vi "Mike.vi"() -> ()   [LabVIEW 2013]
uses:
  <vilib>/Analysis/2dsp.llb/Real FFT.vi
  <instrlib>/niUSRP/niUSRP Fetch Rx Data (CDB).vi
  <vilib>/Analysis/NI_AALPro.lvlib
panel:
  out "Waveform Graph 3":dbl[](graph)
  out "Waveform Graph 2":dbl[][](graph)
  out "Waveform Graph":dbl[](graph)
  in  "stop":bool
  in  "RX number of samples":i64=100000
  out "RX coerced gain":dbl format="%#_6f"
  out "RX coerced IQ rate":dbl=100000.0 format="%#_6p"
  in  "RX gain":dbl format="%#_6f"
  in  "RX IQ rate":dbl=100000.0 format="%#_6p"
  in  "device names":refnum<k15>
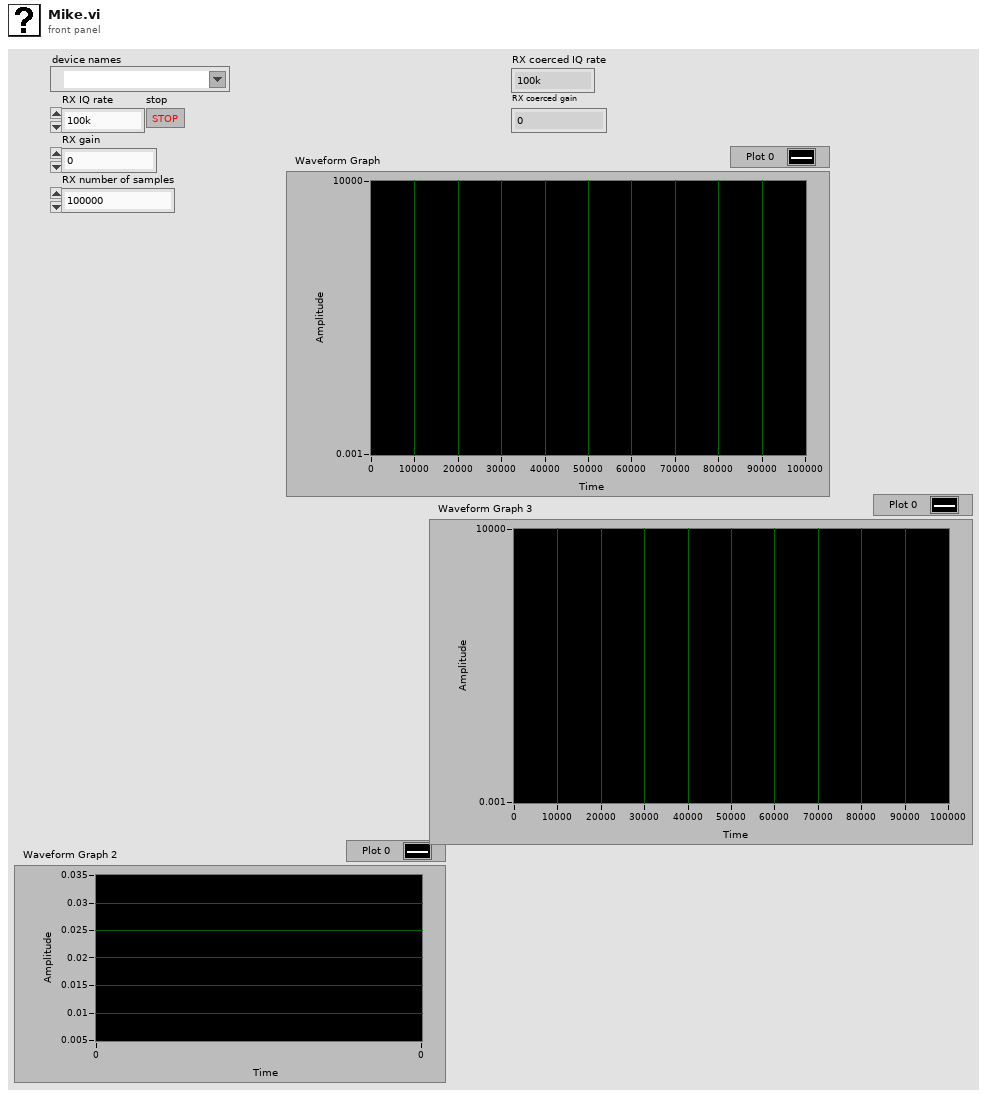
[diagram p1: front panel]
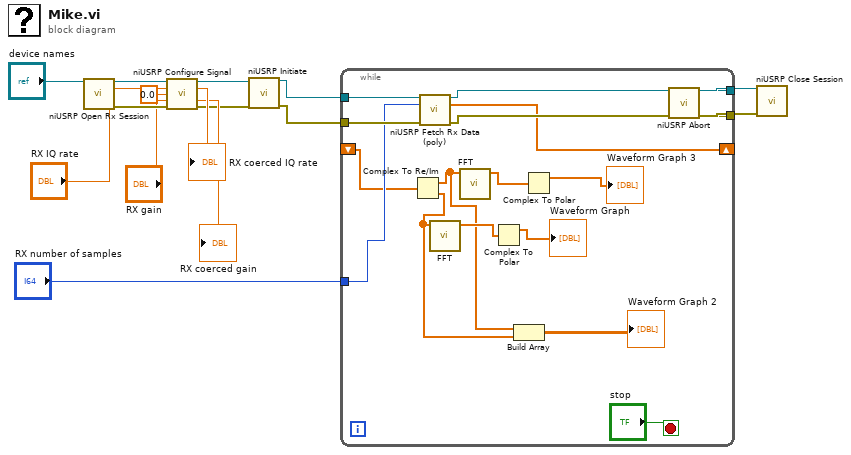
[diagram p0: block diagram]
diagram:
  n1 = call <instrlib>:"niUSRP Open Rx Session.vi"("device names"="device names") -> ("session handle out"=w16:refnum<k15>, "error out"=w14:errorcluster)  [unwired: 13 in]
  n2 = call <instrlib>:"niUSRP Configure Signal.vi"("session handle"=w16, "IQ rate"="RX IQ rate", "carrier frequency"=0.0, "gain"="RX gain", "error in (no error)"=w14) -> ("session handle out"=w3:refnum<k15>, "coerced IQ rate"=→"RX coerced IQ rate":dbl, "coerced gain"=→"RX coerced gain":dbl, "error out"=w2:errorcluster)  [unwired: 6 in, 1 out]
  n3 = call <instrlib>:"niUSRP Initiate.vi"("session handle"=w3, "error in (no error)"=w2) -> ("session handle out"=w4:refnum<k15>, "error out"=w8:errorcluster)  [unwired: 12 in]
  n4 = while {
    tunnel: w4 -> [w32]
    tunnel: w8 -> [w31]
    tunnel: [w30] -> w7
    tunnel: [w29] -> w6
    tunnel: "RX number of samples" -> [w26]
    shift-right: [w27] -> _
    shift-left: _ -> [w23]
    stop <- "stop" stop-if-true
    n5 = Complex To Re/Im(x + iy=w23) -> (x=w21:dbl[], y=w20:dbl[])
    n6 = call-poly <instrlib>:"niUSRP Fetch Rx Data (poly).vi"("session handle"=w32, "number of samples"=w26, "error in (no error)"=w31) -> ("session handle out"=w30:refnum<k15>, "data"=w27:cdb[], "error out"=w29:errorcluster)  [unwired: 9 in, 1 out]
    n7 = call-poly <vilib>:"FFT.vi"("X"=w20) -> ("FFT {X}"=w25:cdb[])  [unwired: 9 in, 1 out]
    n8 = call-poly <vilib>:"FFT.vi"("X"=w21) -> ("FFT {X}"=w22:cdb[])  [unwired: 9 in, 1 out]
    n9 = Complex To Polar(r * e^(i*theta)=w25) -> (r=→"Waveform Graph":dbl[])  [unwired: 1 out]
    n10 = Build Array(w21, w20) -> (→"Waveform Graph 2":dbl[][])
    n11 = Complex To Polar(r * e^(i*theta)=w22) -> (r=→"Waveform Graph 3":dbl[])  [unwired: 1 out]
  }
  n12 = call <instrlib>:"niUSRP Abort.vi"("session handle"=w7, "error in (no error)"=w6) -> ("session handle out"=w15:refnum<k15>, "error out"=w13:errorcluster)  [unwired: 12 in]
  n13 = call <instrlib>:"niUSRP Close Session.vi"("session handle"=w15, "error in (no error)"=w13) -> ()  [unwired: 13 in, 1 out]
